vi "Module Top Level.vi"(8 "error in":errorcluster, 11 "FPGA Ref":T1) -> (0 "error out":errorcluster)   [LabVIEW 2018, in "Inputs.lvlib"]
doc: "This is the top level VI for this module. It uses a queue for communications and is stopped user a user event. The general architecture is similar to a simple queued message handler.\n\nThe VIs associated with this module are organized in a LabVIEW Library."
uses:
  Inputs.lvlib
  FPGA/FPGA VI Reference.ctl
  Private Controls/Host Comms Data.ctl
  Private Controls/Module Data.ctl
  Private Controls/Module Action.ctl
  Top Level/Shared Controls/Acq Data.ctl
  <vilib>/Utility/error.llb/Error Cluster From Error Code.vi
  <vilib>/rvi/errors/niLvFpgaAdjustHostInterfaceError.vi
  <vilib>/rvi/interface/nirviReadWriteControl/nirviReadWriteControl.xnode
  RT-UDP Writer/UDP Writer.lvlib
  <vilib>/ptbypt/NI_PtbyPt.lvlib
  NiFpgaLv.dll
  <vilib>/rvi/interface/Simulation/niFpgaSimulationCallBeginRW.vi
panel:
  # "Inputs"
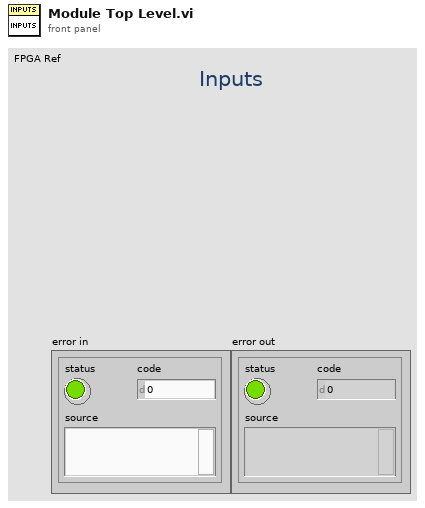
[diagram p1: front panel]
types:
  T1 = typedef "FPGA VI Reference.ctl" = refnum<k20>
  T2 = typedef "Inputs.lvlib/Host Comms Data.ctl" = cluster{"FPGA Ref":T1}
  T3 = typedef "Acq Data.ctl" = cluster{"00-00-9220":dbl[], "00-01-9220":dbl[], "02-02-9219":dbl[], "02-03-9227":dbl[], "02-05-9205":dbl[]}
  T4 = typedef "Inputs.lvlib/Module Data.ctl" = cluster{"Data":variant, "Action":T5}
  T5 = typedef "Inputs.lvlib/Module Action.ctl" = enum16{"Init", "RPMs", "Temps", "AI", "Timeout", "Error"}
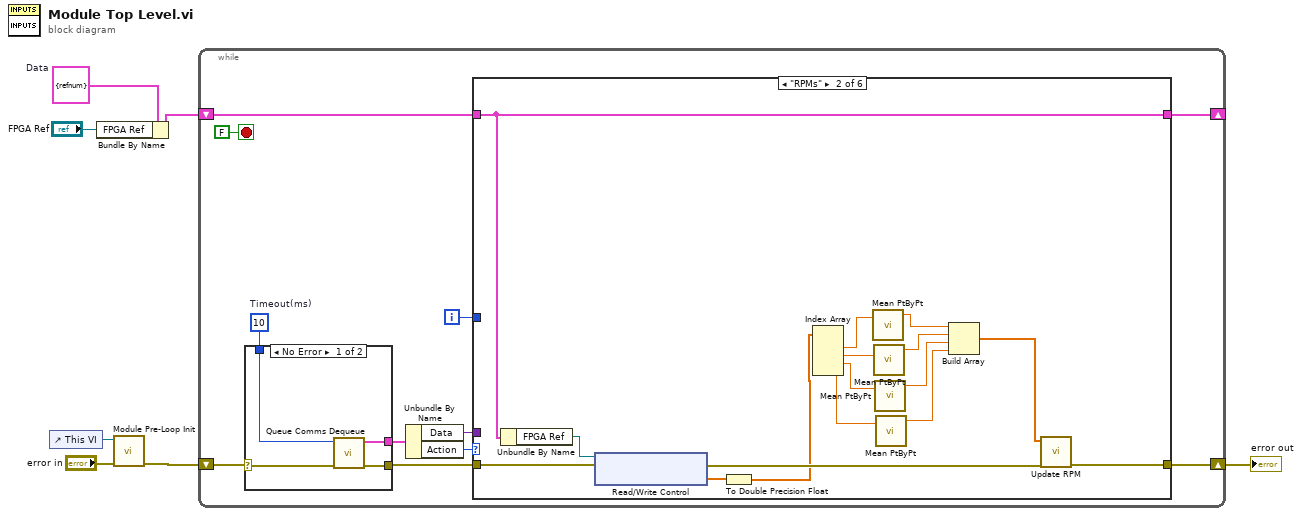
[diagram p0: block diagram]
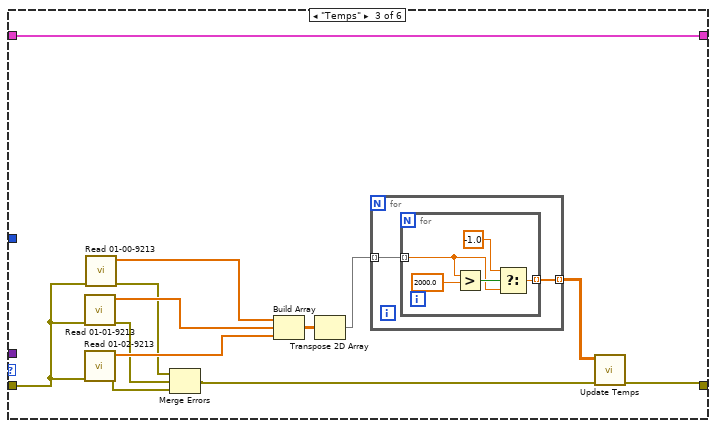
[diagram p3: hidden frame]
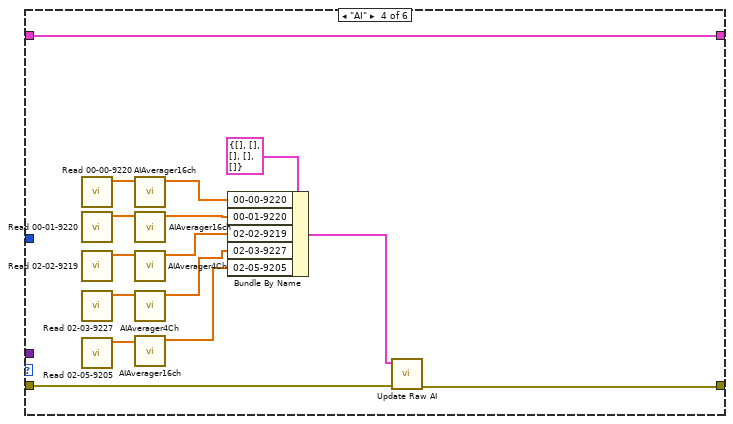
[diagram p4: hidden frame]
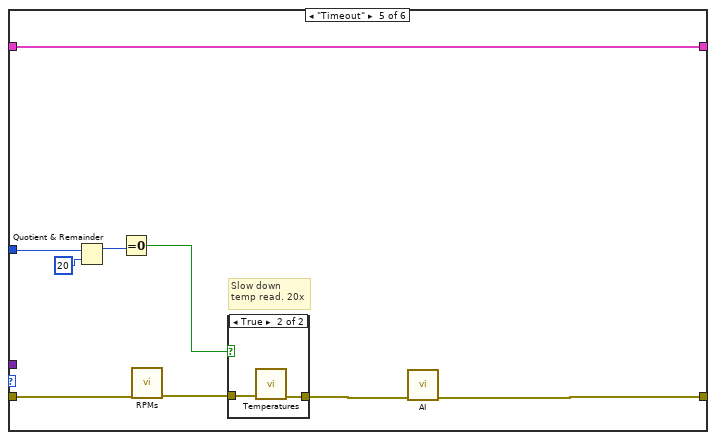
[diagram p5: hidden frame]
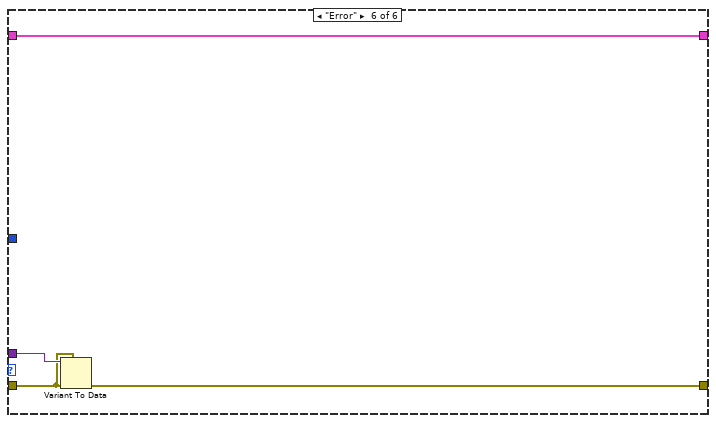
[diagram p7: hidden frame]
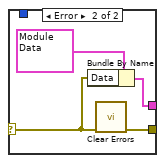
[diagram p8: hidden frame]
diagram:
  w4 = T2 {"FPGA Ref"=refnum}  # Data
  n1 = control-ref of="This VI"() -> (w7:refnum<vi>)
  n2 = Bundle By Name(cluster=w4, "FPGA Ref"="FPGA Ref") -> (w2:T2)
  n3 = call "Module Pre-Loop Init.vi"("error in (no error)"="error in", "Top Level VI Ref in"=w7) -> ("error out"=w3:errorcluster)  [unwired: 9 in]
  n4 = while {
    shift-right: [w14] -> w5
    shift-left: w3 -> [w13]
    shift-right: [w12] -> _
    shift-left: w2 -> [w11]
    i -> [w9]
    stop <- FALSE stop-if-true
    w8 = 10  # Timeout(ms)
    n5 = case shown="No Error" w13 {
      selector: w13 -> [w90 w93]
      tunnel: [w91 w94] -> w18
      tunnel: [w89 w92] -> w15
      tunnel: w8 -> [w88 _]
      frame No Error {
        n6 = call "Queue Comms Dequeue.vi"("error in (no error)"=w90, "Timeout(ms)"=w88) -> ("error out"=w89:errorcluster, "element"=w91:T4)  [unwired: 8 in]
      }
      frame Error {
        n7 = Bundle By Name(cluster=T4 {"Data"=variant, "Action"=enum."Error"} ("element"), "Data"=w93) -> (w94:T4)
        n8 = call <vilib>:"Clear Errors.vi"("error in (no error)"=w93) -> ("error out"=w92:errorcluster)  [unwired: 5 in, 1 out]
      }
    }
    n9 = Unbundle By Name(w18) -> ("Data"=w16:variant, "Action"=w17:T5)
    n10 = case shown="\"RPMs\"" w17 {
      tunnel: w16 -> [_ _ _ _ _ w87]
      tunnel: w15 -> [w20 w36 w41 w70 w79 w86]
      tunnel: [w20 w32 w44 w69 w76 w85] -> w14
      tunnel: [w19 w35 w49 w71 w80 w84] -> w12
      tunnel: w11 -> [w19 w35 w49 w71 w80 w84]
      tunnel: w9 -> [_ _ _ _ w75 _]
      frame "Init" {
      }
      frame "RPMs" {
        n11 = Unbundle By Name(w35) -> ("FPGA Ref"=w34:T1)
        n12 = xnode "Read/Write Control"("FPGA VI Reference In"=w34, "error in"=w36) -> ("error out"=w33:errorcluster, "00-03-9402 (RPM)"=w22:sgl[])  [unwired: 1 out]
        n13 = To Double Precision Float(number=w22) -> (double precision float=w21:dbl[])
        n14 = Index Array(array=w21) -> (element #1=w31:dbl, element #2=w29:dbl, element #3=w28:dbl, element #4=w27:dbl)  [unwired: 4 in]
        n15 = call <vilib>:"Mean PtByPt.vi"("x"=w31) -> ("mean"=w30:dbl)  [unwired: 3 in, 1 out]
        n16 = call <vilib>:"Mean PtByPt.vi"("x"=w29) -> ("mean"=w26:dbl)  [unwired: 3 in, 1 out]
        n17 = call <vilib>:"Mean PtByPt.vi"("x"=w28) -> ("mean"=w25:dbl)  [unwired: 3 in, 1 out]
        n18 = call <vilib>:"Mean PtByPt.vi"("x"=w27) -> ("mean"=w24:dbl)  [unwired: 3 in, 1 out]
        n19 = Build Array(w30, w26, w25, w24) -> (w23:dbl[])
        n20 = call "Update RPM.vi"("error in"=w33, "RPMs"=w23) -> ("error out"=w32:errorcluster)  [unwired: 9 in]
      }
      frame "Temps" {
        n21 = call "Read 01-01-9213.vi"("error in"=w41) -> ("error out"=w39:errorcluster, "01-01-9213"=w47:dbl[])  [unwired: 9 in]
        n22 = call "Read 01-02-9213.vi"("error in"=w41) -> ("error out"=w40:errorcluster, "01-02-9213"=w46:dbl[])  [unwired: 9 in]
        n23 = call "Read 01-00-9213.vi"("error in"=w41) -> ("error out"=w38:errorcluster, "01-00-9213"=w48:dbl[])  [unwired: 9 in]
        n24 = Merge Errors(w38, w39, w40) -> (w37:errorcluster)
        n25 = Build Array(w48, w47, w46) -> (w45:dbl[][])
        n26 = Transpose 2D Array(2D array=w45) -> (transposed array=w43:dbl[][])
        n27 = for {
          tunnel: w43 -> [w51] mode=indexing
          tunnel: [w50] -> w42 mode=indexing
          n28 = for {
            tunnel: w51 -> [w54] mode=indexing
            tunnel: [w52] -> w50 mode=indexing
            n29 = Greater?(x=w54, y=2000.0) -> (0:w55:bool)
            n30 = Select(t=-1.0, s=w55, f=w54) -> (s? t:f=w52:dbl)
          }
        }
        n31 = call "Update Temps.vi"("error in"=w37, "Temps"=w42) -> ("error out"=w44:errorcluster)  [unwired: 9 in]
      }
      frame "AI" {
        n32 = call "Read 00-00-9220.vi"() -> ("00-00-9220"=w66:dbl[])  [unwired: 11 in]
        n33 = call "Read 00-01-9220.vi"() -> ("00-01-9220"=w64:dbl[])  [unwired: 11 in]
        n34 = call "Read 02-02-9219.vi"() -> ("02-02-9219"=w60:dbl[])  [unwired: 11 in]
        n35 = call "Read 02-03-9227.vi"() -> ("02-03-9227"=w58:dbl[])  [unwired: 11 in]
        n36 = call "Read 02-05-9205.vi"() -> ("02-05-9205"=w63:dbl[])  [unwired: 11 in]
        n37 = call "AIAverager16ch.vi"("Array in"=w66) -> ("Array out"=w65:dbl[])  [unwired: 10 in]
        n38 = call "AIAverager16ch.vi"("Array in"=w64) -> ("Array out"=w61:dbl[])  [unwired: 10 in]
        n39 = call "AIAverager4Ch.vi"("Array in"=w60) -> ("Array out"=w59:dbl[])  [unwired: 10 in]
        n40 = call "AIAverager4Ch.vi"("Array in"=w58) -> ("Array out"=w57:dbl[])  [unwired: 10 in]
        n41 = call "AIAverager16ch.vi"("Array in"=w63) -> ("Array out"=w62:dbl[])  [unwired: 10 in]
        n42 = Bundle By Name(cluster=T3 {"00-00-9220"=[], "00-01-9220"=[], "02-02-9219"=[], "02-03-9227"=[], "02-05-9205"=[]} ("Raw AI"), "00-00-9220"=w65, "00-01-9220"=w61, "02-02-9219"=w59, "02-03-9227"=w57, "02-05-9205"=w62) -> (w67:T3)
        n43 = call "Update Raw AI.vi"("error in"=w70, "AI"=w67) -> ("error out"=w69:errorcluster)  [unwired: 9 in]
      }
      frame "Timeout" {
        # "Slow down \ntemp read. 20x"
        n44 = Quotient & Remainder(x=w75, y=20) -> (x-y*floor(x/y)=w73:i32)  [unwired: 1 out]
        n45 = Equal To 0?(x=w73) -> (x = 0?=w72:bool)
        n46 = call "RPMs.vi"("error in"=w79) -> ("error out"=w78:errorcluster)  [unwired: 10 in]
        n47 = case shown="True" w72 {
          tunnel: w78 -> [w81 w83]
          tunnel: [w81 w82] -> w77
          frame False {
          }
          frame True {
            n48 = call "Temperatures.vi"("error in"=w83) -> ("error out"=w82:errorcluster)  [unwired: 10 in]
          }
        }
        n49 = call "AI.vi"("error in"=w77) -> ("error out"=w76:errorcluster)  [unwired: 10 in]
      }
      frame "Error" {
        n50 = Variant To Data(error in=w86, type=w86, Variant=w87) -> (error out=w85:errorcluster)  [unwired: 1 out]
      }
    }
  }
  "error out" <- w5
